vi "Transform2ToDiff.vi"(1 "End Transform":T1, 2 "Start Transform":T1) -> (0 "Differential":dbl[](array[numeric]))   [LabVIEW 2017, in "NI_Kinematics.lvlib"]
uses:
  <vilib>/robotics/Kinematics/NI_Kinematics.lvlib
  <vilib>/Analysis/Matrix/Datatypes/RealMatrix.ctl
  <vilib>/Analysis/NI_AALPro.lvlib
  <vilib>/Analysis/Matrix/NI_Matrix.lvlib
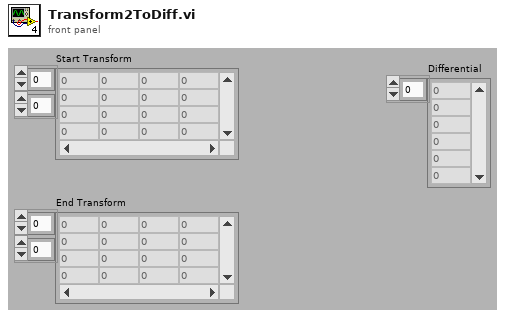
[diagram p1: front panel]
types:
  T1 = typedef "NI_Matrix.lvlib/RealMatrix.ctl" = dbl[][]
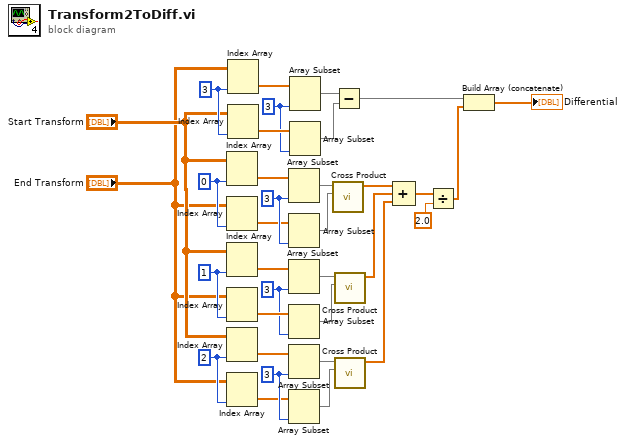
[diagram p0: block diagram]
diagram:
  w20 = 3 ("length")
  w19 = 2 ("disabled index (col)")
  w21 = 3 ("length")
  w22 = 1 ("disabled index (col)")
  w28 = 3 ("length")
  w27 = 0 ("disabled index (col)")
  w29 = 3 ("length")
  w30 = 3 ("disabled index (col)")
  n1 = Index Array(array="Start Transform", index (col)=w27) -> (element=w25:dbl[])  [unwired: 1 in]
  n2 = Index Array(array="End Transform", index (col)=w27) -> (element=w26:dbl[])  [unwired: 1 in]
  n3 = Index Array(array="Start Transform", index (col)=w22) -> (element=w24:dbl[])  [unwired: 1 in]
  n4 = Index Array(array="End Transform", index (col)=w22) -> (element=w23:dbl[])  [unwired: 1 in]
  n5 = Index Array(array="Start Transform", index (col)=w19) -> (element=w17:dbl[])  [unwired: 1 in]
  n6 = Index Array(array="End Transform", index (col)=w19) -> (element=w18:dbl[])  [unwired: 1 in]
  n7 = Index Array(array="End Transform", index (col)=w30) -> (element=w34:dbl[])  [unwired: 1 in]
  n8 = Index Array(array="Start Transform", index (col)=w30) -> (element=w33:dbl[])  [unwired: 1 in]
  n9 = Array Subset(array=w25, length=w28) -> (w2:dbl[])  [unwired: 1 in]
  n10 = Array Subset(array=w26, length=w28) -> (w3:dbl[])  [unwired: 1 in]
  n11 = Array Subset(array=w24, length=w21) -> (w6:dbl[])  [unwired: 1 in]
  n12 = Array Subset(array=w23, length=w21) -> (w5:dbl[])  [unwired: 1 in]
  n13 = Array Subset(array=w17, length=w20) -> (w8:dbl[])  [unwired: 1 in]
  n14 = Array Subset(array=w18, length=w20) -> (w9:dbl[])  [unwired: 1 in]
  n15 = Array Subset(array=w34, length=w29) -> (w32:dbl[])  [unwired: 1 in]
  n16 = Array Subset(array=w33, length=w29) -> (w31:dbl[])  [unwired: 1 in]
  n17 = call <vilib>:"Cross Product.vi"("B Vector"=w3, "A Vector"=w2) -> ("Cross Product"=w1:dbl[])  [unwired: 8 in, 1 out]
  n18 = Subtract(x=w32, y=w31) -> (x-y=w16:dbl[])
  n19 = call <vilib>:"Cross Product.vi"("B Vector"=w5, "A Vector"=w6) -> ("Cross Product"=w4:dbl[])  [unwired: 8 in, 1 out]
  n20 = call <vilib>:"Cross Product.vi"("B Vector"=w9, "A Vector"=w8) -> ("Cross Product"=w7:dbl[])  [unwired: 8 in, 1 out]
  n21 = Compound Arithmetic op=ADD(w1, w4, w7) -> (w15:dbl[])
  n22 = Divide(x=w15, y=2.0) -> (x/y=w14:dbl[])
  n23 = Build Array (concatenate)(w16, w14) -> (→"Differential":dbl[])
